vi "Read configuration.vi"(8 "error in":errorcluster, 11 "CEF_serializable node folder in":refnum<class "CEF_serializable node folder.lvclass">) -> (0 "error out":errorcluster, 2 "cfg":refnum<class "CEF_serializable node folder configuration.lvclass">, 3 "CEF_serializable node folder out":refnum<class "CEF_serializable node folder.lvclass">)   [LabVIEW 2023, in "CEF_serializable node folder.lvclass"]
doc: "Copyright 2017 National Instruments Corporation\n\nLicensed under the Apache License, Version 2.0 (the \"License\"); you may not use this file except in compliance with the License. You may obtain a copy of the License at http://www.apache.org/licenses/LICENSE-2.0\nUnless required by applicable law or agreed to in writing, software distributed under the License is distributed on an \"AS IS\" BASIS, WITHOUT WARRANTIES OR CONDITIONS OF ANY KIND, either express or implied. See the License for the specific language governing permissions and limitations under the License."
uses:
  CEF_serializable node folder.lvclass
  CEF_serializable node folder.lvclass/CEF_serializable node folder.ctl
  folder configuration/CEF_serializable node folder configuration.lvclass
  C:/ProgramData/CORE/W80-4/HW Config/VI Packages/Configuration Framework/serializable configuration/NISE_CEF_serializable configuration.lvclass
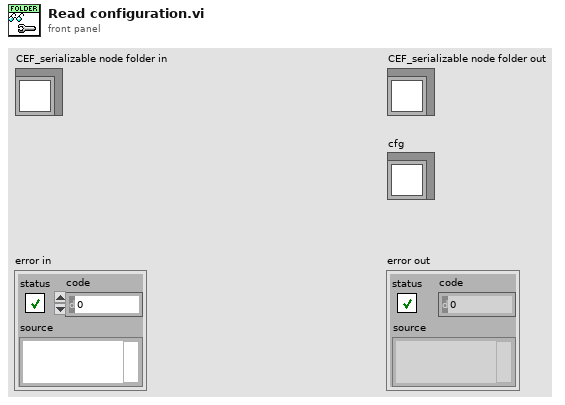
[diagram p1: front panel]
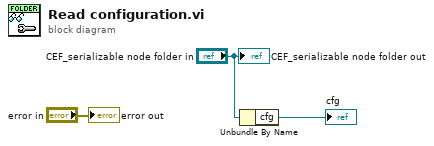
[diagram p0: block diagram]
diagram:
  n1 = Unbundle By Name("CEF_serializable node folder in") -> ("cfg"=→"cfg":refnum<class "CEF_serializable node folder configuration.lvclass">)
  "error out" <- "error in"
  "CEF_serializable node folder out" <- "CEF_serializable node folder in"
